vi "Write Area.vi"(8 "error in (no error)":errorcluster, 10 "Area":dbl, 11 "Figure in":refnum<class "Figure.lvclass">) -> (0 "error out":errorcluster, 3 "Figure out":refnum<class "Figure.lvclass">)   [LabVIEW 2021, in "Figure.lvclass"]
uses:
  Figure.lvclass
  Figure.lvclass/Figure.ctl
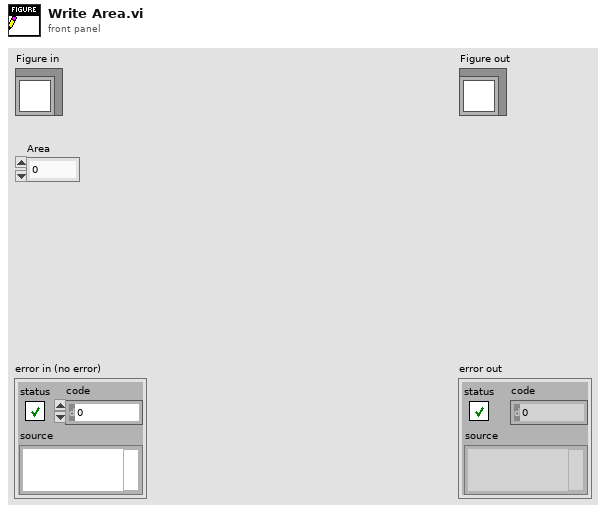
[diagram p1: front panel]
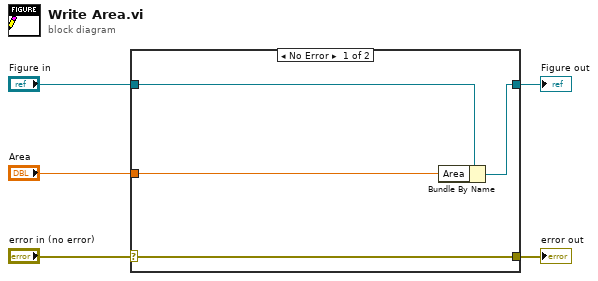
[diagram p0: block diagram]
diagram:
  n1 = case shown="No Error" "error in (no error)" {
    selector: "error in (no error)" -> [w9 w10]
    tunnel: [w9 w10] -> w4
    tunnel: [w7 w11] -> w2
    tunnel: "Figure in" -> [w8 w11]
    tunnel: "Area" -> [w6 _]
    frame No Error {
      n2 = Bundle By Name(cluster=w8, "Area"=w6) -> (w7:refnum<class "Figure.lvclass">)
    }
    frame Error {
    }
  }
  "error out" <- w4
  "Figure out" <- w2
